vi "PH_AxisGUI_NF.contents.vi"   [LabVIEW 2014, in "PH_AxisGUI_NF.lvlib"]
doc: "This class is forseen to control up to three New Focus motors (class: NF87xx).\n\nThis class is part of the PHELIX user layer."
uses:
  PH_AxisGUI_NF.lvlib
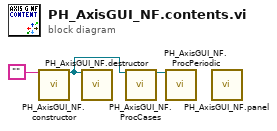
[diagram p0: block diagram]
diagram:
  n1 = call "PH_AxisGUI_NF.constructor.vi"("name"="") -> ("i ref out"=w1:refnum<vi>)  [unwired: 16 in, 2 out]
  n2 = call "PH_AxisGUI_NF.destructor.vi"("i ref in"=w1) -> ()  [unwired: 18 in, 1 out]
  n3 = call "PH_AxisGUI_NF.ProcCases.vi"("i ref in"=w1) -> ("i ref out"=w3:refnum<vi>)  [unwired: 16 in, 2 out]
  n4 = call "PH_AxisGUI_NF.ProcPeriodic.vi"("i ref in"=w3) -> ()  [unwired: 16 in, 3 out]
  n5 = call "PH_AxisGUI_NF.panel.vi"() -> ()  [unwired: 19 in, 1 out]
